vi "Adjust Splitter.vi"(8 "error in":errorcluster, 10 "Show":bool, 11 "Bottom Panel in":refnum<class "RightDock.lvclass">) -> (0 "error out":errorcluster, 3 "Bottom Panel out":refnum<class "RightDock.lvclass">)   [LabVIEW 2023, in "Docking.lvlib" / "RightDock.lvclass"]
doc: "This class is designed so that ancestor classes can rescale the UI to fit the actor core of the ancestor UI."
uses:
  RightDock.lvclass
  C:/Users/Public/Documents/Development/builds/Framework/Engine.lvlibp/Engine/Library/Engine.lvclass
  C:/Users/Public/Documents/Development/Application/Docking/Panels/Docking/Docking.lvclass
  Docking/Docking.lvclass/Docking.ctl
  Docking/Read Splitter Refnum.vi
  Docking/Read InitialPosition.vi
  builds/Framework/Engine.lvlibp/Engine/Accessors/Read VI Ref.vi
  builds/Framework/Engine.lvlibp/Engine/Library/Engine.lvclass
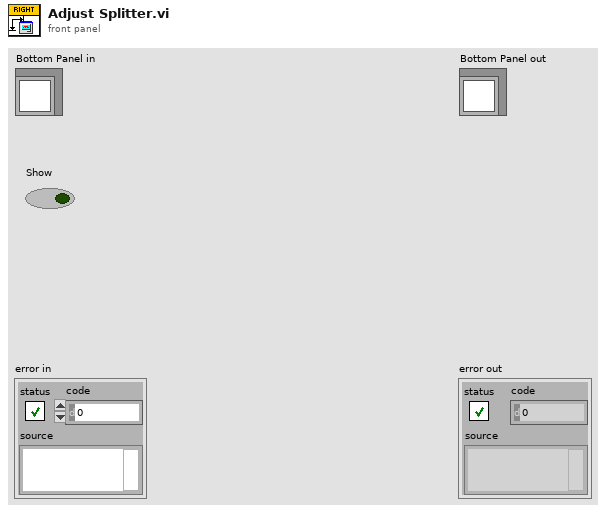
[diagram p1: front panel]
types:
  T1 = typedef "LVPointTypeDef.ctl" = cluster{"Horizontal":i16, "Vertical":i16}
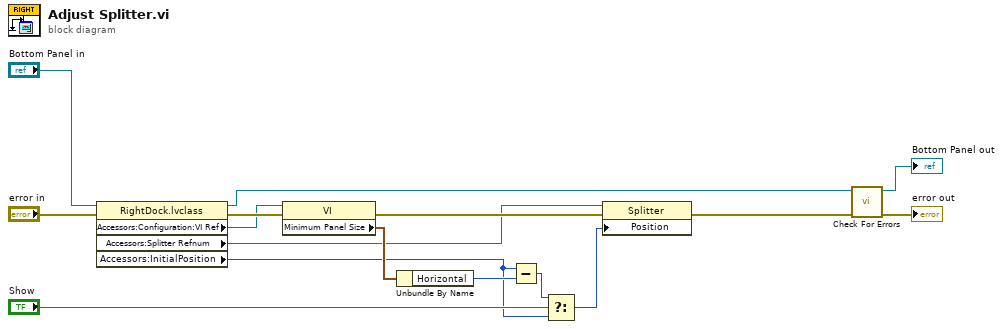
[diagram p0: block diagram]
diagram:
  n1 = property class="RightDock.lvclass"(reference="Bottom Panel in", error in="error in") -> (reference out=w8:refnum<class "RightDock.lvclass">, error out=w14:errorcluster, "Accessors:Configuration:VI Ref"=w4:refnum<vi>, "Accessors:Splitter Refnum"=w3:refnum<vi>, "Accessors:InitialPosition"=w1:i32)
  n2 = property class="VI"(reference=w4, error in=w14) -> (error out=w9:errorcluster, "Minimum Panel Size"=w13:T1)  [unwired: 1 out]
  n3 = Unbundle By Name(w13) -> ("Horizontal"=w2:i16)
  n4 = Subtract(x=w1, y=w2) -> (x-y=w12:i32)
  n5 = Select(t=w12, s="Show", f=w1) -> (s? t:f=w10:i32)
  n6 = property class="Splitter"(reference=w3, error in=w9, "Position"=w10) -> (error out=w6:errorcluster)  [unwired: 1 out]
  n7 = call "Check For Errors.vi"("error in"=w6, "Engine in"=w8) -> ("error out"=→"error out":errorcluster, "Engine out"=→"Bottom Panel out":refnum<class "RightDock.lvclass">)  [unwired: 8 in]
